vi "Switchboard.vi"(11 "Input parameters":T1={"Measurement type"=enum."Test", "Sensor type"=enum."HPK_6in_135", "Identifier"="test.txt", "Open after execution?"=FALSE, "Plot after execution?"=FALSE, "Display channel"=0, "Voltage Delay (s)"=0.5, "Switch Delay (s)"=0.01, "VISA resource name source"="", "VISA resource name DMM"="", "VISA resource name LCR"="", "Compliance  Level (uA)"=10.0, "Voltage Limit (V)"=1000.0, "Data storage location"="", "Scan voltages"="", "Use source as DMM?"=FALSE, "Single channel?"=FALSE} {"Voltage Limit (V)" format="%#_13g"; "Voltage Delay (s)" format="%#_13g"; "Switch Delay (s)" format="%#_13g"}) -> (3 "Output config":i32[](array[numeric]))   [LabVIEW 2016]
uses:
  Input_parameters.ctl
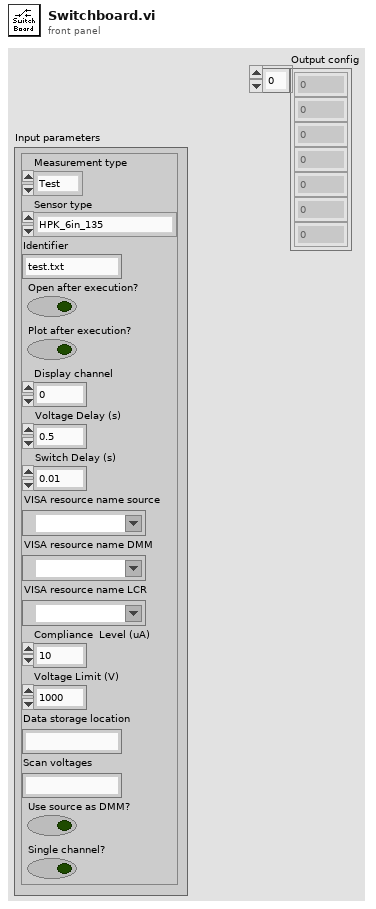
[diagram p1: front panel]
types:
  T1 = typedef "Input_parameters.ctl" = cluster{"Measurement type":enum16{"IV", "CV", "Test"}, "Sensor type":enum16{"HPK_6in_135", "HPK_8in_256", "INF_8in_256", "Diode"}, "Identifier":string, "Open after execution?":bool, "Plot after execution?":bool, "Display channel":i32, "Voltage Delay (s)":dbl, "Switch Delay (s)":dbl, "VISA resource name source":refnum<visa-resource-name>, "VISA resource name DMM":refnum<visa-resource-name>, "VISA resource name LCR":refnum<visa-resource-name>, "Compliance  Level (uA)":dbl, "Voltage Limit (V)":dbl, "Data storage location":string, "Scan voltages":string, "Use source as DMM?":bool, "Single channel?":bool}
  T2 = enum16{"HPK_6in_135", "HPK_8in_256", "INF_8in_256", "Diode"}
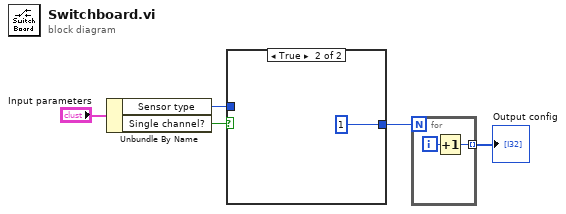
[diagram p0: block diagram]
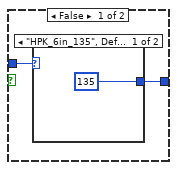
[diagram p2: hidden frame]
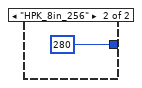
[diagram p3: hidden frame]
diagram:
  n1 = Unbundle By Name("Input parameters") -> ("Sensor type"=w1:T2, "Single channel?"=w3:bool)
  n2 = case shown="True" w3 {
    tunnel: [w6 1] -> w2
    tunnel: w1 -> [w7 _]
    frame False {
      n3 = case shown="\"HPK_6in_135\", Default" w7 {
        tunnel: [135 280] -> w6
        frame "HPK_6in_135", Default {
        }
        frame "HPK_8in_256" {
        }
      }
    }
    frame True {
    }
  }
  n4 = for {
    N: w2 -> [_]
    tunnel: [w11] -> w5 mode=indexing
    i -> [w12]
    n5 = Increment(x=w12) -> (x+1=w11:i32)
  }
  "Output config" <- w5
